vi "SPOL_temps_PB3.vi"() -> ()   [LabVIEW 2009]
uses:
  <vilib>/Utility/file.llb/Read From Spreadsheet File (string).vi
panel:
  in  "stop":bool
  in  "Select":bool
  in  "Plot":bool
  out "Housekeeping File":path caption="selected path"
  out "SPOL ATE Temperatures":T1(graph)
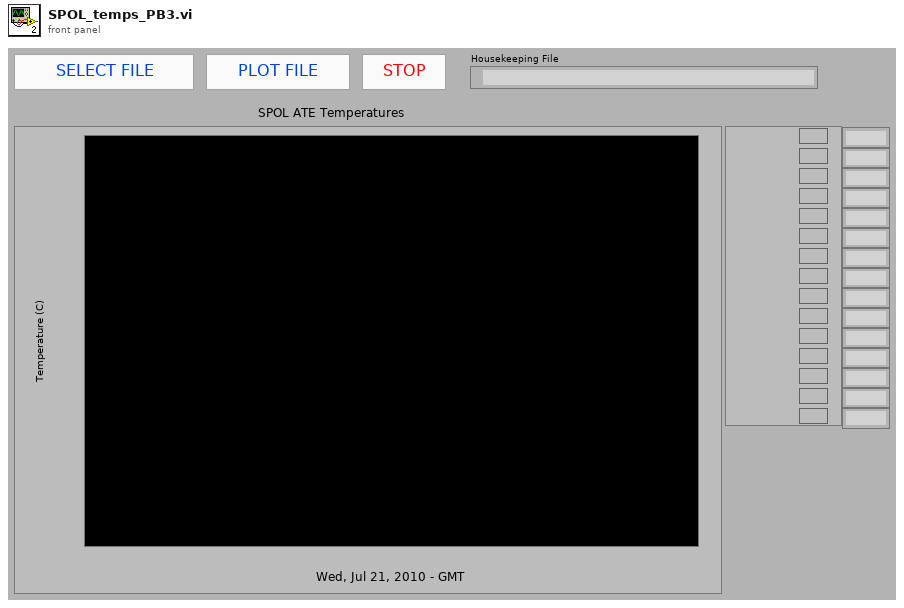
[diagram p1: front panel]
types:
  T1 = cluster{"[0]":dbl, "[1]":dbl, "[2]":dbl, "[3]":dbl, "[4]":dbl, "[5]":dbl, "[6]":dbl, "[7]":dbl, "[8]":dbl, "[9]":dbl, "[10]":dbl, "[11]":dbl, "[12]":dbl, "[13]":dbl, "[14]":dbl}
  T2 = cluster{"[0]":dbl, "[1]":dbl, "[2]":dbl, "[3]":dbl, "[4]":dbl, "[5]":dbl, "[6]":dbl, "[7]":dbl, "[8]":dbl, "[9]":dbl, "[10]":dbl, "[11]":dbl, "[12]":dbl, "[13]":dbl, "[14]":dbl}[]
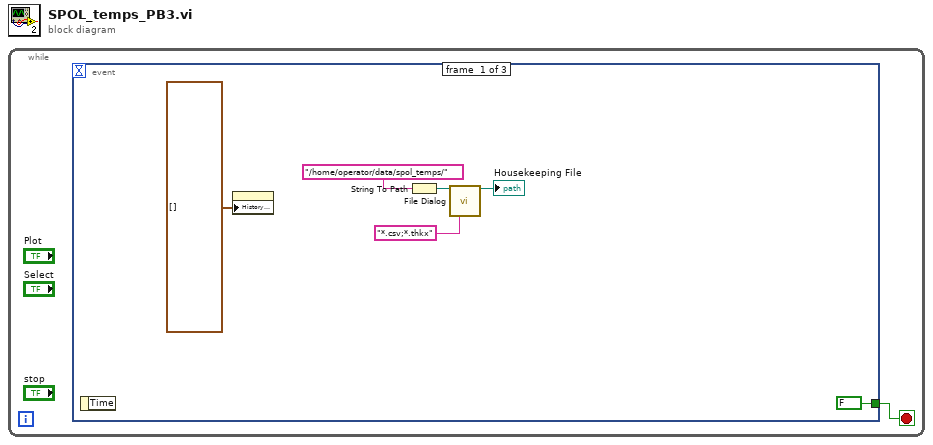
[diagram p0: block diagram]
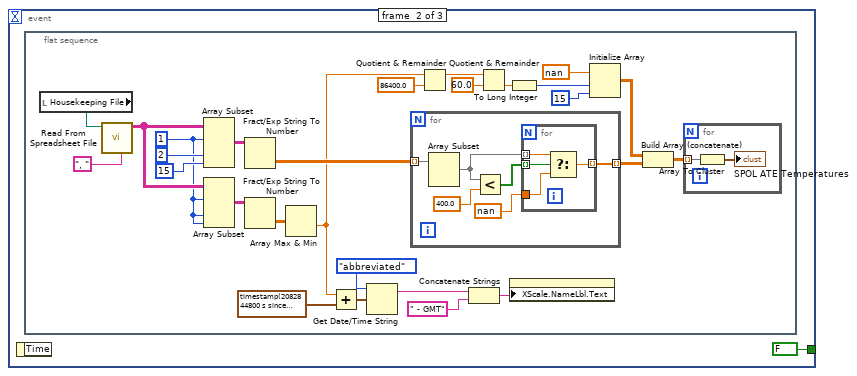
[diagram p2: hidden frame]
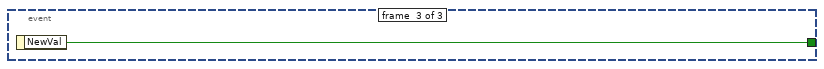
[diagram p3: hidden frame]
diagram:
  n1 = while {
    stop <- w1 stop-if-true
    n2 = event shown="[1] \"Plot\": Value Change" {
      selector: _ -> [_ _ _]
      dyn-events: _ -> [_ _ _]
      timeout: _ -> [_ _ _]
      tunnel: [FALSE ("NewVal") FALSE w48] -> w1
      event #0 {
        n3 = event-data() -> ()  [unwired: 1 in, 1 out]
        n4 = property on="SPOL ATE Temperatures" class="WFChart (strict)"("History Data"=T2 []) -> ()  [unwired: 2 in, 2 out]
        n5 = String To Path(string="/home/operator/data/spol_temps/") -> (path=w5:path)
        n6 = call "File Dialog"("start path"=w5, "pattern (all files)"="*.csv;*.thkx") -> ("selected path"=→"Housekeeping File":path)  [unwired: 10 in, 3 out]
      }
      event #1 {
        n7 = event-data() -> ()  [unwired: 1 in, 1 out]
        n8 = flat-sequence {
          frame #0 {
            w28 = 1 ("index")
            n9 = local read "Housekeeping File"() -> (w35:path)
            n10 = call-poly <vilib>:"Read From Spreadsheet File.vi"("delimiter (\\t)"=", " ("delimiter (\\t)"), "file path (dialog if empty)"=w35) -> ("all rows"=w32:string[][])  [unwired: 5 in, 4 out]
            n11 = Array Subset(array=w32, index (row)=w28, index (col)=2 ("index"), length (col)=15 ("length")) -> (w21:string[][])  [unwired: 1 in]
            n12 = Array Subset(array=w32, index (row)=w28, index (col)=w28, length (col)=w28) -> (w31:string[][])  [unwired: 1 in]
            n13 = Fract/Exp String To Number(string=w21) -> (number=w33:dbl[][])  [unwired: 3 in, 1 out]
            n14 = Fract/Exp String To Number(string=w31) -> (number=w18:dbl[][])  [unwired: 3 in, 1 out]
            n15 = Array Max & Min(array=w18) -> (min value=w13:dbl)  [unwired: 3 out]
            n16 = Add(x=w13, y=timestamp(2082844800 s since 1904-01-01)) -> (x+y=w26:timestamp)
            n17 = Get Date/Time String(date format (0)=enum16{"short", "long", "abbreviated"}."abbreviated", seconds (now)=w26) -> (date string=w25:string)  [unwired: 1 in, 1 out]
            n18 = for {
              tunnel: w33 -> [w39] mode=indexing
              tunnel: [w38] -> w9 mode=indexing
              n19 = Array Subset(array=w39) -> (w42:dbl[])  [unwired: 2 in]
              n20 = Less?(x=w42, y=400.0 ("element")) -> (x < y?=w41:bool[])
              n21 = for {
                tunnel: w41 -> [w47] mode=indexing
                tunnel: w42 -> [w45] mode=indexing
                tunnel: nan ("number/path/refnum") -> [w46]
                tunnel: [w44] -> w38 mode=indexing
                n22 = Select(t=w45, s=w47, f=w46) -> (s? t:f=w44:dbl)
              }
            }
            n23 = Quotient & Remainder(x=w13, y=86400.0) -> (x-y*floor(x/y)=w14:dbl)  [unwired: 1 out]
            n24 = Concatenate Strings(w25, " - GMT" ("string")) -> (w24:string)
            n25 = Quotient & Remainder(x=w14, y=60.0) -> (floor(x/y)=w17:dbl)  [unwired: 1 out]
            n26 = To Long Integer(number=w17) -> (32bit integer=w12:i32)
            n27 = property on="SPOL ATE Temperatures" class="WFChart (strict)"("XScale.NameLbl.Text"=w24) -> ()  [unwired: 2 in, 2 out]
            n28 = Initialize Array(nan ("element"), w12, 15 ("dimension size")) -> (w11:dbl[][])
            n29 = Build Array (concatenate)(w11, w9) -> (w10:dbl[][])
            n30 = for {
              tunnel: w10 -> [w37] mode=indexing
              n31 = Array To Cluster(array=w37) -> (cluster=→"SPOL ATE Temperatures":T1)
            }
          }
        }
      }
      event #2 {
        n32 = event-data() -> ("NewVal"=w48:bool)  [unwired: 1 in]
      }
    }
  }
